vi "Test Pixy2 Functionality.vi"() -> ()   [LabVIEW 2018]
uses:
  source/library/Types/Intersection.ctl
  source/library/Types/Vector.ctl
  source/library/Types/Block.ctl
  <vilib>/Rock Robotics/SystemInterfaces/i2clib/i2c_bus.ctl
  source/library/Interface/Pixy Com.lvclass
  source/deviceSupport/FRC/I2C/RoboRIO I2C.lvclass
  source/library/Pixy2.lvlib
  <vilib>/Rock Robotics/SystemInterfaces/spilib/spi_bus.ctl
  source/deviceSupport/FRC/SPI/RoboRIO SPI.lvclass
  source/deviceSupport/FRC/UART/RoboRIO UART.lvclass
  <vilib>/Rock Robotics/WPI/SerialPort/WPI_SerialPort.ctl
panel:
  out "Index":i32
  out "blocks":T1[](array[typedef])
  out "fps":u32
  out "Line vectors":T2[](array[typedef])
  out "intersections":T3[](array[typedef])
  out "view":picture
  in  "Stop Button":bool
  in  "message":T4(tab)
  in  "color":cluster{"r":u8, "g":u8, "b":u8}
  in  "lamp enable":cluster{"upper":bool, "lower":bool}
  in  "signature map":u8=255 format="%.0x"
  in  "max blocks":u8=255
  in  "features":enum16{"Main Features", "All Features"}(ring)
  in  "feature map":u8=7 format="%.0x"
  in  "mode":u8 format="%.0x"
  in  "vector":u8
  out "Color":u32(colorbox)
  in  "saturate?":bool
  in  "y":u16 max=207
  in  "x":u16 max=315
  in  "brightness":u8
  out "error out":errorcluster
  in  "send":bool
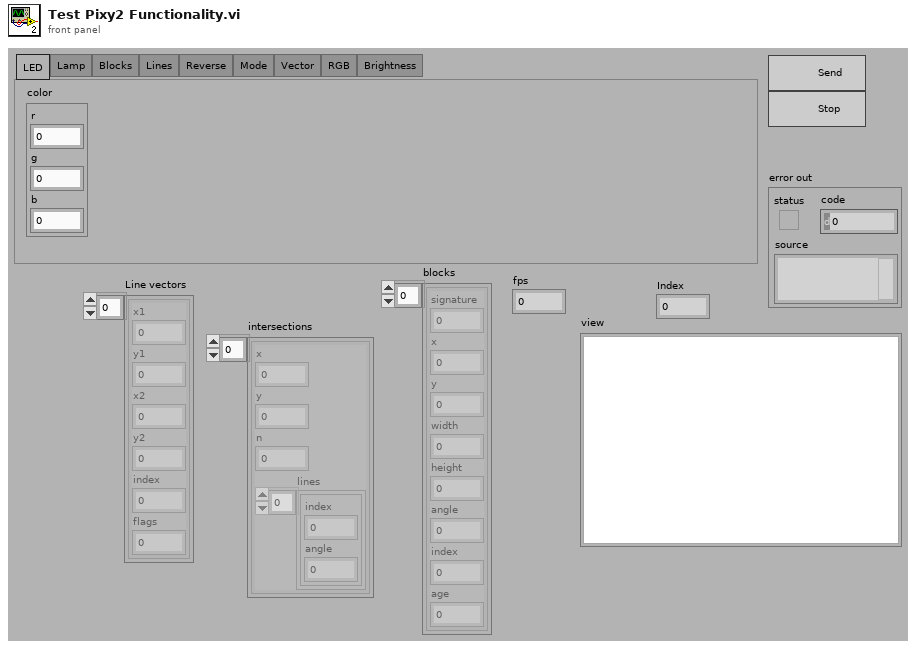
[diagram p1: front panel]
types:
  T1 = typedef "Pixy2.lvlib/Block.ctl" = cluster{"signature":u16, "x":u16, "y":u16, "width":u16, "height":u16, "angle":i16, "index":u8, "age":u8}
  T2 = typedef "Pixy2.lvlib/Vector.ctl" = cluster{"x1":u8, "y1":u8, "x2":u8, "y2":u8, "index":u8, "flags":u8}
  T3 = typedef "Pixy2.lvlib/Intersection.ctl" = cluster{"x":u8, "y":u8, "n":u8, "lines":cluster{"index":u8, "angle":i16}[]}
  T4 = enum32{"LED", "Lamp", "Blocks", "Lines", "Reverse", "Mode", "Vector", "RGB", "Brightness"}
  T5 = typedef "i2c_bus.ctl" = enum16{"I2C On-Board", "I2C MXP", "Invalid"}
  T6 = typedef "spi_bus.ctl" = enum16{"SPI On-Board, CS0", "SPI On-Board, CS1", "SPI On-Board, CS2", "SPI On-Board, CS3", "SPI MXP", "Invalid"}
  T7 = typedef "WPI_SerialPort.ctl" = enum16{"Onboard RS-232", "MXP TTL", "USB 1", "USB 2"}
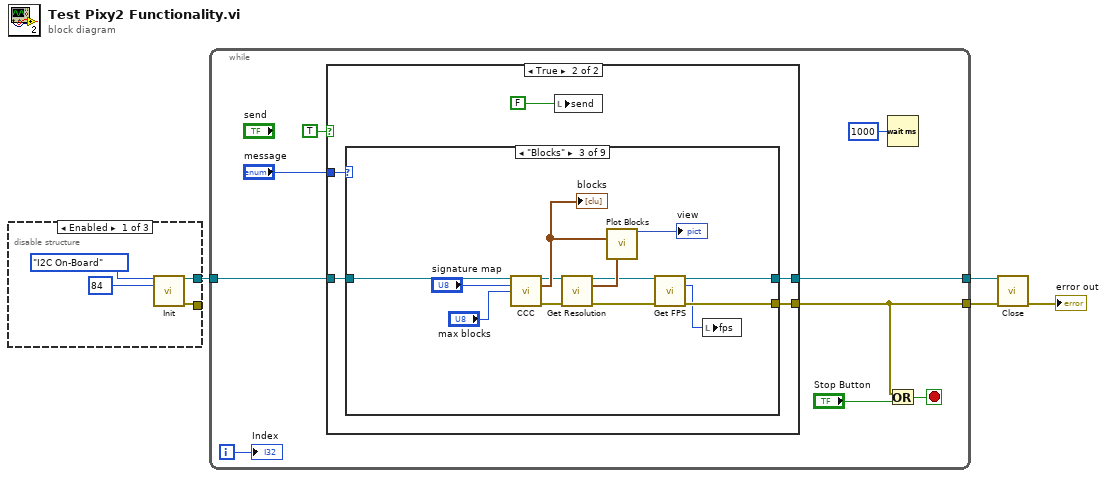
[diagram p0: block diagram]
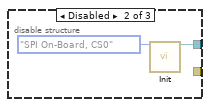
[diagram p2: hidden frame]
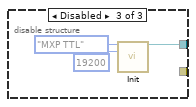
[diagram p3: hidden frame]
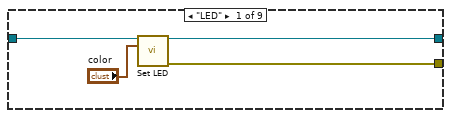
[diagram p5: hidden frame]
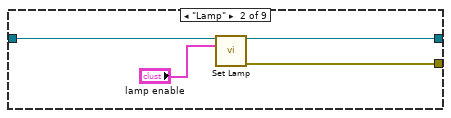
[diagram p6: hidden frame]
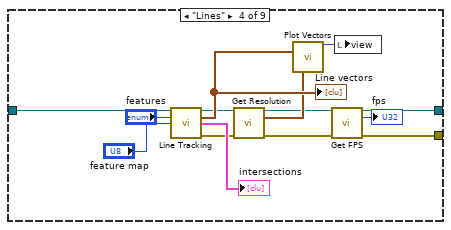
[diagram p7: hidden frame]
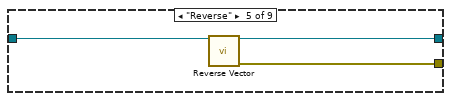
[diagram p8: hidden frame]
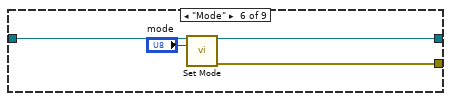
[diagram p9: hidden frame]
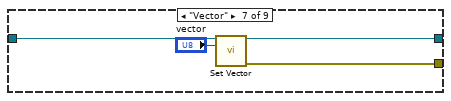
[diagram p10: hidden frame]
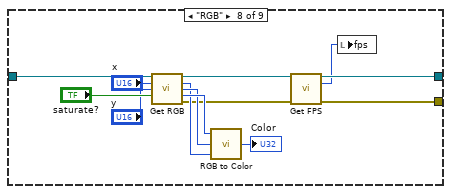
[diagram p11: hidden frame]
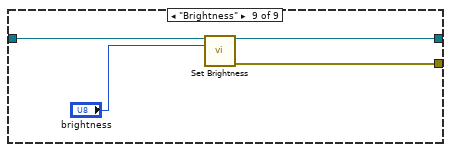
[diagram p12: hidden frame]
diagram:
  n1 = disable-structure shown="Enabled" {
    disable-tunnel: [w8 w10 w13] -> w4
    disable-tunnel: [w5 _ _] -> _
    frame Enabled {
      n2 = call "Init.vi"("I2C bus"=i2c_bus."I2C On-Board" ("I2C Bus"), "device address"=u8 84 ("Device Address")) -> ("comm interface out"=w8:refnum<class "Pixy Com.lvclass">, "error out"=w5:errorcluster)  [unwired: 12 in]
    }
    frame Disabled {
      n3 = call "Init.vi"("SPI Bus"=spi_bus."SPI On-Board, CS0") -> ("comm interface out"=w10:refnum<class "Pixy Com.lvclass">)  [unwired: 13 in, 1 out]
    }
    frame Disabled {
      n4 = call "Init.vi"("serial port"=WPI_SerialPort."MXP TTL", "baud rate"=u32 19200) -> ("comm interface out"=w13:refnum<class "Pixy Com.lvclass">)  [unwired: 12 in, 1 out]
    }
  }
  n5 = while {
    tunnel: w4 -> [w22]
    tunnel: [w20] -> w3
    tunnel: [w21] -> w2
    i -> [w14]
    stop <- w19 stop-if-true
    n6 = case shown="True" TRUE {
      tunnel: w22 -> [w23 w27]
      tunnel: [_ w25] -> w20
      tunnel: [w23 w26] -> w21
      tunnel: "message" -> [_ w24]
      frame False {
      }
      frame True {
        n7 = case shown="\"Blocks\"" w24 {
          tunnel: w27 -> [w32 w36 w49 w63 w66 w70 w74 w87 w90]
          tunnel: [w31 w35 w38 w52 w65 w69 w73 w76 w89] -> w26
          tunnel: [w30 w33 w39 w51 w64 w68 w72 w78 w88] -> w25
          frame "LED" {
            n8 = call "Set LED.vi"("comm interface in"=w32, "color"="color") -> ("comm interface out"=w31:refnum<class "Pixy Com.lvclass">, "error out"=w30:errorcluster)  [unwired: 12 in]
          }
          frame "Lamp" {
            n9 = call "Set Lamp.vi"("comm interface in"=w36, "lamp enable"="lamp enable") -> ("comm interface out"=w35:refnum<class "Pixy Com.lvclass">, "error out"=w33:errorcluster)  [unwired: 12 in]
          }
          frame "Blocks" {
            n10 = call "CCC.vi"("comm interface in"=w49, "signature map"="signature map", "max blocks"="max blocks") -> ("comm interface out"=w44:refnum<class "Pixy Com.lvclass">, "blocks"=w46:T1[], "error out"=w43:errorcluster)  [unwired: 10 in]
            "blocks" <- w46
            n11 = call "Get Resolution.vi"("comm interface in"=w44, "error in"=w43) -> ("comm interface out"=w41:refnum<class "Pixy Com.lvclass">, "resolution"=w42:cluster{"width":u16, "height":u16}, "error out"=w40:errorcluster)  [unwired: 11 in]
            n12 = call "Plot Blocks.vi"("blocks"=w46, "pixy resolution"=w42) -> ("picture out"=→"view":picture)  [unwired: 13 in]
            n13 = call "Get FPS.vi"("comm interface in"=w41, "error in"=w40) -> ("comm interface out"=w38:refnum<class "Pixy Com.lvclass">, "fps"=w37:u32, "error out"=w39:errorcluster)  [unwired: 11 in]
            n14 = local write "fps"(w37) -> ()
          }
          frame "Lines" {
            n15 = call "Line Tracking.vi"("comm interface in"=w63, "features"="features", "feature map"="feature map") -> ("comm interface out"=w57:refnum<class "Pixy Com.lvclass">, "vectors"=w60:T2[], "intersections"=→"intersections":T3[], "error out"=w56:errorcluster)  [unwired: 8 in, 1 out]
            "Line vectors" <- w60
            n16 = call "Get Resolution.vi"("comm interface in"=w57, "error in"=w56) -> ("comm interface out"=w54:refnum<class "Pixy Com.lvclass">, "resolution"=w55:cluster{"width":u16, "height":u16}, "error out"=w53:errorcluster)  [unwired: 11 in]
            n17 = call "Plot Vectors.vi"("vectors"=w60, "pixy resolution"=w55) -> ("picture out"=w59:picture)  [unwired: 13 in]
            n18 = call "Get FPS.vi"("comm interface in"=w54, "error in"=w53) -> ("comm interface out"=w52:refnum<class "Pixy Com.lvclass">, "fps"=→"fps":u32, "error out"=w51:errorcluster)  [unwired: 11 in]
            n19 = local write "view"(w59) -> ()
          }
          frame "Reverse" {
            n20 = call "Reverse Vector.vi"("comm interface in"=w66) -> ("comm interface out"=w65:refnum<class "Pixy Com.lvclass">, "error out"=w64:errorcluster)  [unwired: 13 in]
          }
          frame "Mode" {
            n21 = call "Set Mode.vi"("comm interface in"=w70, "mode"="mode") -> ("comm interface out"=w69:refnum<class "Pixy Com.lvclass">, "error out"=w68:errorcluster)  [unwired: 12 in]
          }
          frame "Vector" {
            n22 = call "Set Vector.vi"("comm interface in"=w74, "vector"="vector") -> ("comm interface out"=w73:refnum<class "Pixy Com.lvclass">, "error out"=w72:errorcluster)  [unwired: 12 in]
          }
          frame "RGB" {
            n23 = call "Get RGB.vi"("comm interface in"=w87, "x"="x", "y"="y", "saturate?"="saturate?") -> ("comm interface out"=w77:refnum<class "Pixy Com.lvclass">, "blue"=w83:u8, "green"=w84:u8, "red"=w85:u8, "error out"=w79:errorcluster)  [unwired: 7 in]
            n24 = call <vilib>:"RGB to Color.vi"("B"=w83, "G"=w84, "R"=w85) -> ("Color"=→"Color":u32)
            n25 = call "Get FPS.vi"("comm interface in"=w77, "error in"=w79) -> ("comm interface out"=w76:refnum<class "Pixy Com.lvclass">, "fps"=w75:u32, "error out"=w78:errorcluster)  [unwired: 11 in]
            n26 = local write "fps"(w75) -> ()
          }
          frame "Brightness" {
            n27 = call "Set Brightness.vi"("comm interface in"=w90, "brightness"="brightness") -> ("comm interface out"=w89:refnum<class "Pixy Com.lvclass">, "error out"=w88:errorcluster)  [unwired: 12 in]
          }
        }
        n28 = local write "send"(FALSE ("send button")) -> ()
      }
    }
    n29 = Wait (ms)(milliseconds to wait=u32 1000) -> ()  [unwired: 1 out]
    n30 = Or(x=w20, y="Stop Button") -> (x .or. y?=w19:bool)
    "Index" <- w14
  }
  n31 = call-dynamic "Close.vi"("comm interface in"=w2, "error in"=w3) -> ("error out"=→"error out":errorcluster)  [unwired: 13 in]
